vi "DAQ 2장 실습 FFT_Sampling Rate Example.vi"() -> ()   [LabVIEW 2021]
uses:
  <vilib>/DAQmx/write.llb/DAQmx Write (Analog 1D DBL 1Chan NSamp).vi
  <vilib>/DAQmx/read.llb/DAQmx Read (Analog Wfm 1Chan NSamp).vi
  <vilib>/DAQmx/create/channels.llb/DAQmx Create Channel (AO-Voltage-Basic).vi
  <vilib>/DAQmx/create/channels.llb/DAQmx Create Channel (AI-Voltage-Basic).vi
  <vilib>/DAQmx/configure/timing.llb/DAQmx Timing (Sample Clock).vi
  <vilib>/DAQmx/miscellaneous.llb/DAQmx Fill In Error Info.vi
  <vilib>/measure/maspectr.llb/FFT Power Spectrum for 1 Chan.vi
  <vilib>/measure/NI_MAPro.lvlib
  <vilib>/Analysis/NI_AALBase.lvlib
  <resource>/objmgr/daqmx.rc
panel:
  in  "DAQmx 디바이스 이름":tag="Dev1"
  in  "아날로그 출력 주파수(Hz)":dbl(knob)=50.0 min=10.0 max=500.0 scale=50.0..500.0
  in  "아날로그 입력 주파수 (Hz)":dbl(knob)=100.0 min=100.0 max=5000.0 scale=100.0..5000.0
  in  "정지":bool
  out "주파수 영역 데이터":cluster{"f0":dbl, "df":dbl, "magnitude":dbl[]}(graph)={"f0"=0.0, "df"=1.0, "magnitude"=[]}
  out "시간 영역 데이터":waveform(dbl)(graph)={"t0"=timestamp(3661848008.3173184 s since 1904-01-01), "dt"=0.01, "Y"=[], "attributes"=variant("NI_ChannelName"=variant(string "Dev2/ai0"), "NI_UnitDescription"=variant(string "Volts"))}
  # "샘플링 속도\n샘플링 속도가 더 크면 클수록 더 정확함 \n데이터 크기가 커짐 (하드웨어의 한계)"
  # "센서 데이터 속도"
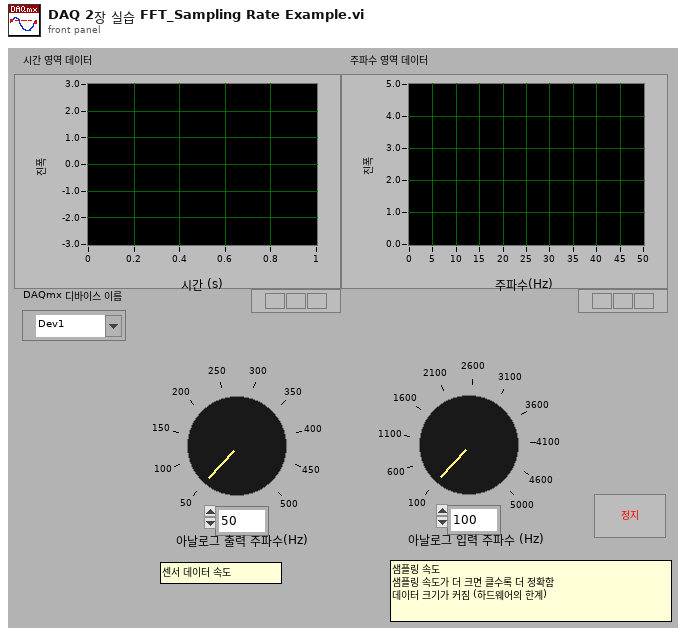
[diagram p1: front panel]
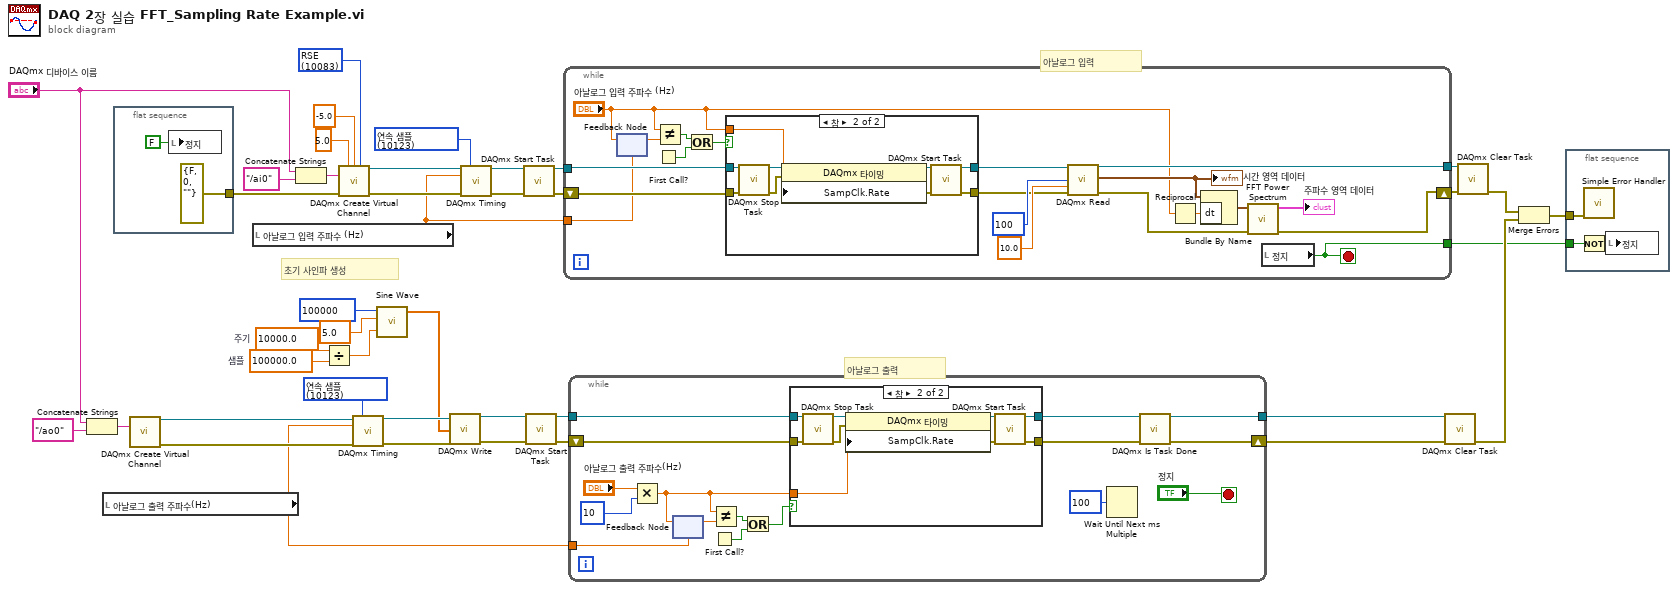
[diagram p0: block diagram]
diagram:
  w1 = 10083 items=["기본"=-1, "RSE"=10083, "NRSE"=10078, "차동"=10106, "유사 차동"=12529] ("input terminal configuration")
  w4 = 10123 items=["유한 샘플"=10178, "연속 샘플"=10123, "하드웨어 타이밍에 의한 단일 포인트"=12522] ("sample mode")
  w5 = 10123 items=["유한 샘플"=10178, "연속 샘플"=10123, "하드웨어 타이밍에 의한 단일 포인트"=12522] ("sample mode")
  w30 = 10000.0  # 주기
  w32 = 100000.0  # 샘플
  # "아날로그 출력"
  # "아날로그 입력"
  # "초기 사인파 생성"
  n1 = Concatenate Strings ("문자열 연결")("DAQmx 디바이스 이름", "/ao0" ("문자열")) -> (w9:string)
  n2 = local read "아날로그 출력 주파수(Hz)"() -> (w2:dbl)
  n3 = flat-sequence {
    tunnel: [cluster{"상태":bool, "코드":i32, "소스":string} {"상태"=FALSE, "코드"=0, "소스"=""} ("에러 입력")] -> w14
    frame #0 {
      n4 = local write "정지"(FALSE ("정지")) -> ()
    }
  }
  n5 = call-poly <vilib>:"DAQmx Create Virtual Channel.vi"("physical channels"=w9) -> ("task out"=w23:refnum<k21>, "error out"=w3:errorcluster)  [unwired: 13 in]
  n6 = local read "아날로그 입력 주파수 (Hz)"() -> (w7:dbl)
  n7 = Concatenate Strings ("문자열 연결")("DAQmx 디바이스 이름", "/ai0" ("문자열")) -> (w11:string)
  n8 = Divide ("나누기")(x=w30, y=w32) -> (x/y=w31:dbl)
  n9 = call-poly <vilib>:"DAQmx Create Virtual Channel.vi"("maximum value"=5.0 ("최대값"), "minimum value"=-5.0 ("최소값"), "input terminal configuration"=w1, "physical channels"=w11, "error in"=w14) -> ("task out"=w39:refnum<k21>, "error out"=w8:errorcluster)  [unwired: 9 in]
  n10 = call-poly <vilib>:"DAQmx Timing.vi"("task/channels in"=w23, "sample mode"=w4, "rate"=w2, "error in"=w3) -> ("task out"=w34:refnum<k21>, "error out"=w33:errorcluster)  [unwired: 10 in]
  n11 = call <vilib>:"Sine Wave.vi"("samples"=100000 ("샘플"), "amplitude"=5.0 ("진폭"), "frequency"=w31) -> ("sine wave"=w27:dbl[])  [unwired: 2 in, 2 out]
  n12 = call-poly <vilib>:"DAQmx Write.vi"("task/channels in"=w34, "data"=w27, "error in"=w33) -> ("task out"=w22:refnum<k21>, "error out"=w21:errorcluster)  [unwired: 10 in, 1 out]
  n13 = call-poly <vilib>:"DAQmx Timing.vi"("task/channels in"=w39, "sample mode"=w5, "rate"=w7, "error in"=w8) -> ("task out"=w24:refnum<k21>, "error out"=w38:errorcluster)  [unwired: 10 in]
  n14 = call <vilib>:"DAQmx Start Task.vi"("task/channels in"=w24, "error in"=w38) -> ("task out"=w37:refnum<k21>, "error out"=w36:errorcluster)  [unwired: 12 in]
  n15 = call <vilib>:"DAQmx Start Task.vi"("task/channels in"=w22, "error in"=w21) -> ("task out"=w26:refnum<k21>, "error out"=w25:errorcluster)  [unwired: 12 in]
  n16 = while {
    tunnel: w37 -> [w54]
    tunnel: [w61] -> w18
    tunnel: w7 -> [w45]
    tunnel: [w44] -> w6
    shift-right: [w60] -> w19
    shift-left: w36 -> [w51]
    stop <- w44 stop-if-true
    n17 = feedback-in #1("아날로그 입력 주파수 (Hz)") -> ()
    n18 = feedback #1(w45) -> (w50:dbl)
    n19 = First Call? ("첫번째 호출?")() -> (First Call?: T/F=w46:bool)
    n20 = Not Equal? ("같지 않음?")(x="아날로그 입력 주파수 (Hz)", y=w50) -> (x != y?=w49:bool)
    n21 = Or(x=w49, y=w46) -> (x .or. y?=w47:bool)
    n22 = case shown="참" w47 {
      tunnel: w54 -> [w65 w70]
      tunnel: w51 -> [w64 w69]
      tunnel: [w65 w68] -> w53
      tunnel: [w64 w67] -> w52
      tunnel: "아날로그 입력 주파수 (Hz)" -> [_ w66]
      frame False {
      }
      frame True {
        n23 = call <vilib>:"DAQmx Stop Task.vi"("task/channels in"=w70, "error in"=w69) -> ("task out"=w72:refnum<k21>, "error out"=w71:errorcluster)  [unwired: 12 in]
        n24 = property on="프로퍼티 노드" class="DAQmx 타이밍"(reference=w72, error in=w71, "SampClk.Rate"=w66) -> (reference out=w74:refnum<k21>, error out=w73:errorcluster)
        n25 = call <vilib>:"DAQmx Start Task.vi"("task/channels in"=w74, "error in"=w73) -> ("task out"=w68:refnum<k21>, "error out"=w67:errorcluster)  [unwired: 12 in]
      }
    }
    n26 = call-poly <vilib>:"DAQmx Read.vi"("task/channels in"=w53, "number of samples per channel"=100 ("채널당 샘플 개수"), "timeout"=10.0 ("타임아웃"), "error in"=w52) -> ("task out"=w61:refnum<k21>, "data"=w58:waveform(dbl), "error out"=w55:errorcluster)  [unwired: 9 in]
    "시간 영역 데이터" <- w58
    n27 = Reciprocal ("역수")(x="아날로그 입력 주파수 (Hz)") -> (1/x=w57:dbl)
    n28 = Bundle By Name ("웨이브폼 만들기")(cluster=w58, "dt"=w57) -> (w56:waveform(dbl))
    n29 = call-poly <vilib>:"FFT Power Spectrum.vi"("error in (no error)"=w55, "time signal"=w56) -> ("error out"=w60:errorcluster, "power spectrum"=→"주파수 영역 데이터":cluster{"f0":dbl, "df":dbl, "magnitude":dbl[]})  [unwired: 6 in, 2 out]
    n30 = local read "정지"() -> (w44:bool)
  }
  n31 = while {
    tunnel: w26 -> [w84]
    shift-right: [w87] -> w35
    shift-left: w25 -> [w83]
    tunnel: [w88] -> w20
    tunnel: w2 -> [w78]
    stop <- "정지" stop-if-true
    n32 = Multiply ("곱하기")(x="아날로그 출력 주파수(Hz)", y=10) -> (x*y=w76:dbl)
    n33 = feedback #2(w78) -> (w80:dbl)
    n34 = feedback-in #2(w76) -> ()
    n35 = First Call? ("첫번째 호출?")() -> (First Call?: T/F=w77:bool)
    n36 = Not Equal? ("같지 않음?")(x=w76, y=w80) -> (x != y?=w79:bool)
    n37 = Or(x=w79, y=w77) -> (x .or. y?=w75:bool)
    n38 = case shown="참" w75 {
      tunnel: w84 -> [w92 w97]
      tunnel: w83 -> [w91 w96]
      tunnel: [w92 w95] -> w82
      tunnel: [w91 w94] -> w81
      tunnel: w76 -> [_ w93]
      frame False {
      }
      frame True {
        n39 = call <vilib>:"DAQmx Stop Task.vi"("task/channels in"=w97, "error in"=w96) -> ("task out"=w99:refnum<k21>, "error out"=w98:errorcluster)  [unwired: 12 in]
        n40 = property on="프로퍼티 노드" class="DAQmx 타이밍"(reference=w99, error in=w98, "SampClk.Rate"=w93) -> (reference out=w101:refnum<k21>, error out=w100:errorcluster)
        n41 = call <vilib>:"DAQmx Start Task.vi"("task/channels in"=w101, "error in"=w100) -> ("task out"=w95:refnum<k21>, "error out"=w94:errorcluster)  [unwired: 12 in]
      }
    }
    n42 = Wait Until Next ms Multiple ("다음 ms 배수까지 기다림")(millisecond multiple=u32 100 ("밀리초 배수")) -> ()  [unwired: 1 out]
    n43 = call <vilib>:"DAQmx Is Task Done.vi"("task/channels in"=w82, "error in"=w81) -> ("task out"=w88:refnum<k21>, "error out"=w87:errorcluster)  [unwired: 11 in, 1 out]
  }
  n44 = call <vilib>:"DAQmx Clear Task.vi"("task in"=w20, "error in"=w35) -> ("error out"=w16:errorcluster)  [unwired: 13 in]
  n45 = call <vilib>:"DAQmx Clear Task.vi"("task in"=w18, "error in"=w19) -> ("error out"=w17:errorcluster)  [unwired: 13 in]
  n46 = Merge Errors ("에러 병합")(w17, w16) -> (w15:errorcluster)
  n47 = flat-sequence {
    tunnel: w15 -> [w104]
    tunnel: w6 -> [w102]
    frame #0 {
      n48 = Not(x=w102) -> (.not. x?=w103:bool)
      n49 = call <vilib>:"Simple Error Handler.vi"("error in (no error)"=w104) -> ()  [unwired: 4 in, 5 out]
      n50 = local write "정지"(w103) -> ()
    }
  }
